vi "GaussianFitEB.vi"(0 "X":ext[](array[numeric])=[-2.0, -1.0, 0.0, 1.0, 2.0, 3.0] format="%.2e", 7 "Y":ext[](array[numeric])=[17.0, 6.0, 1.0, 2.0, 9.0, 22.0] format="%.2e", 11 "DY":ext[](array[numeric])=[1.0, 1.0, 1.0, 1.0, 1.0, 1.0] format="%.2e") -> (3 "sigma":dbl format="%.2f", 4 "delta sigma rms":dbl format="%.2f", 6 "m":dbl format="%.2f", 8 "delta m rms":dbl format="%.2f", 10 "A":dbl format="%.2f", 13 "Chi square":ext=13.257575757575757575 format="%.4e", 14 "Degrees of freedom":i32=3, 15 "delta A rms":dbl format="%.2f")   [LabVIEW 2014]
panel:
  out "mi":ext[](array[numeric])=[1.378787878787861, -1.77272727272727, 2.621212121212123] format="%.4e"
  out "Error Matrix":dbl[][](array[numeric])=[[0.3606060606060606, 0.03636363636363638, -0.060606060606060656], [0.036363636363636424, 0.3818181818181819, -0.13636363636363638], [-0.06060606060606063, -0.13636363636363638, 0.060606060606060615]] format="%.4e"
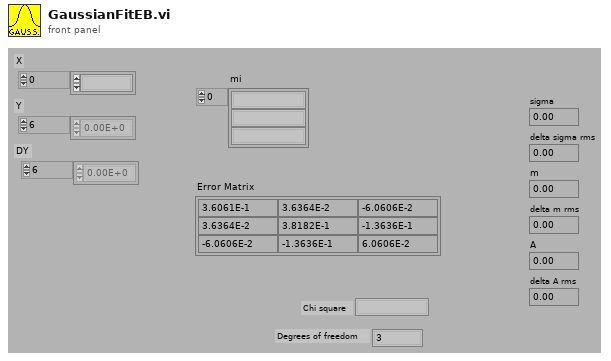
[diagram p1: front panel]
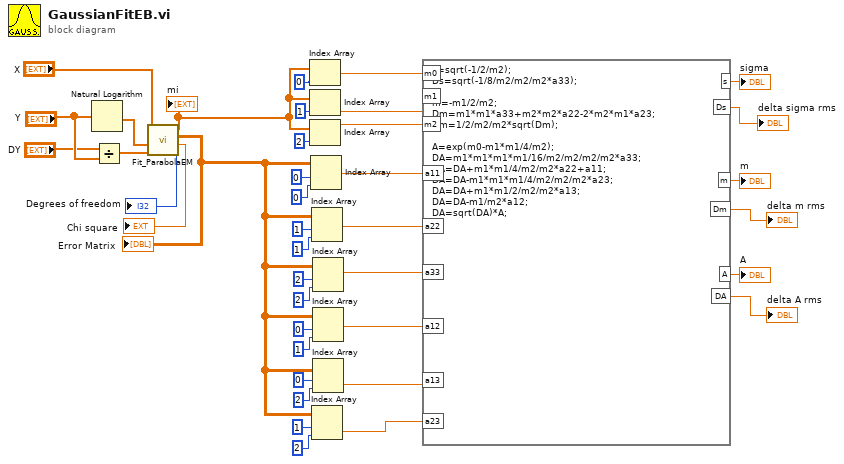
[diagram p0: block diagram]
diagram:
  n1 = Natural Logarithm(1:"Y") -> (0:w19:ext[])
  n2 = Divide(x="DY", y="Y") -> (x/y=w16:ext[])
  n3 = call "Fit_ParabolaEM.vi"("DY"=w16, "Y"=w19, "X"="X") -> ("Degrees of freedom"=→"Degrees of freedom":i32, "Chi square"=→"Chi square":ext, "Error Matrix"=w36:dbl[][], "m"=w37:ext[])  [unwired: 3 in]
  "Error Matrix" <- w36
  "mi" <- w37
  n4 = Index Array(array=w37, index=0 ("Index")) -> (element=w15:ext)
  n5 = Index Array(array=w37, index=1 ("Index")) -> (element=w14:ext)
  n6 = Index Array(array=w37, index=2 ("Index")) -> (element=w13:ext)
  n7 = Index Array(array=w36, index (row)=0 ("Index"), index (col)=0 ("Index")) -> (element=w12:dbl)
  n8 = Index Array(array=w36, index (row)=1 ("Index"), index (col)=1 ("Index")) -> (element=w11:dbl)
  n9 = Index Array(array=w36, index (row)=1 ("Index"), index (col)=2 ("Index")) -> (element=w7:dbl)
  n10 = Index Array(array=w36, index (row)=2 ("Index"), index (col)=2 ("Index")) -> (element=w10:dbl)
  n11 = Index Array(array=w36, index (row)=0 ("Index"), index (col)=1 ("Index")) -> (element=w9:dbl)
  n12 = Index Array(array=w36, index (row)=0 ("Index"), index (col)=2 ("Index")) -> (element=w8:dbl)
  n13 = formula code="s=sqrt(-1/2/m2);\nDs=sqrt(-1/8/m2/m2/m2*a33);\n\nm=-m1/2/m2;\nDm=m1*m1*a33+m2*m2*a22-2*m2*m1*a23;\nDm=1/2/m2/m2*sqrt(Dm);\n\nA=exp(m0-m1*m1/4/m2);\nDA=m1*m1*m1*m1/16/m2/m2/m2/m2*a33;\nDA=DA+m1*m1/4/m2/m2*a22+a11;\nDA=DA-m1*m1*m1/4/m2/m2/m2*a23;\nDA=DA+m1*m1/2/m2/m2*a13;\nDA=DA-m1/m2*a12;\nDA=sqrt(DA)*A;"("m0"=w15, "m1"=w14, "m2"=w13, "a11"=w12, "a22"=w11, "a33"=w10, "a12"=w9, "a13"=w8, "a23"=w7) -> ("s"=→"sigma":dbl, "Ds"=→"delta sigma rms":dbl, "m"=→"m":dbl, "Dm"=→"delta m rms":dbl, "A"=→"A":dbl, "DA"=→"delta A rms":dbl)
